vi "Axis-Angle rotation.vi"(1 "Input vector3":dbl[](array[numeric]), 2 "Rotation axis (UNIT vector3)":dbl[](array[numeric]), 3 "Rotation angle (rad)":dbl) -> (0 "Output vector3":dbl[](array[numeric]))   [LabVIEW 2017]
uses:
  <vilib>/Analysis/baseanly.llb/Real Dot Product.vi
  <vilib>/Analysis/NI_AALBase.lvlib
  <vilib>/Analysis/NI_AALPro.lvlib
panel:
  # "Axis of rotation must be a unit vector."
  # "Rotation is anti-clockwise looking into the axis of rotation."
  # "PN 23/03/18"
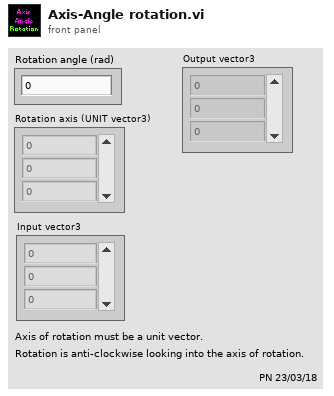
[diagram p1: front panel]
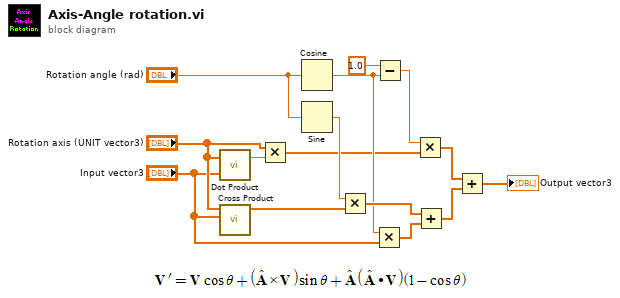
[diagram p0: block diagram]
diagram:
  n1 = call-poly <vilib>:"Dot Product.vi"("Y Vector"="Input vector3", "X Vector"="Rotation axis (UNIT vector3)") -> ("X * Y"=w6:dbl)  [unwired: 1 out]
  n2 = call <vilib>:"Cross Product.vi"("B Vector"="Input vector3", "A Vector"="Rotation axis (UNIT vector3)") -> ("Cross Product"=w15:dbl[])  [unwired: 8 in, 1 out]
  n3 = Multiply(x="Rotation axis (UNIT vector3)", y=w6) -> (x*y=w8:dbl[])
  n4 = Cosine(x="Rotation angle (rad)") -> (cos(x)=w10:dbl)
  n5 = Sine(x="Rotation angle (rad)") -> (sin(x)=w9:dbl)
  n6 = Multiply(x=w9, y=w15) -> (x*y=w12:dbl[])
  n7 = Multiply(x=w10, y="Input vector3") -> (x*y=w11:dbl[])
  n8 = Subtract(x=1.0, y=w10) -> (x-y=w7:dbl)
  n9 = Multiply(x=w7, y=w8) -> (x*y=w14:dbl[])
  n10 = Add(x=w12, y=w11) -> (x+y=w13:dbl[])
  n11 = Add(x=w14, y=w13) -> (x+y=→"Output vector3":dbl[])
